vi "Integral timescale and std errors_PN.vi"(0 "uv_bar (m/s)^2":dbl, 1 "Cross-correlation function":dbl[](array[numeric]), 5 "u2v2_bar (m/s)^4":dbl, 7 "T_meas (s)":dbl, 9 "dt (s)":dbl, 11 "integral cut-off":dbl, 12 "integral post-mult":dbl=1.0, 13 "Multiplyer of Timescale to get Independant samples":dbl=2.0) -> (4 "N independent samples":i32, 6 "Integral timescale (s)":dbl, 10 "Std. err in U (m/s)":dbl, 15 "Std. err in uv (m/s^2)":dbl)   [LabVIEW 2016]
uses:
  <vilib>/Analysis/2dsp.llb/Integral Method.ctl
  <vilib>/Analysis/8numeric.llb/1D Numeric Integration.vi
  <vilib>/Analysis/NI_AALPro.lvlib
panel:
  out "Normalised cross-correlation function up to cut-offs":cluster{dbl, "dt (s)":dbl, "Rxy":dbl[]}(graph)
  out "Cross-correlation function (positive signed)":cluster{dbl, "dt (s)":dbl, "Rxy":dbl[]}(graph)
  # "SE_mean is only meaningful in autocorrelation  (i.e. with U = V)"
  # "PN 06/01/2011,\n      01/12/2016"
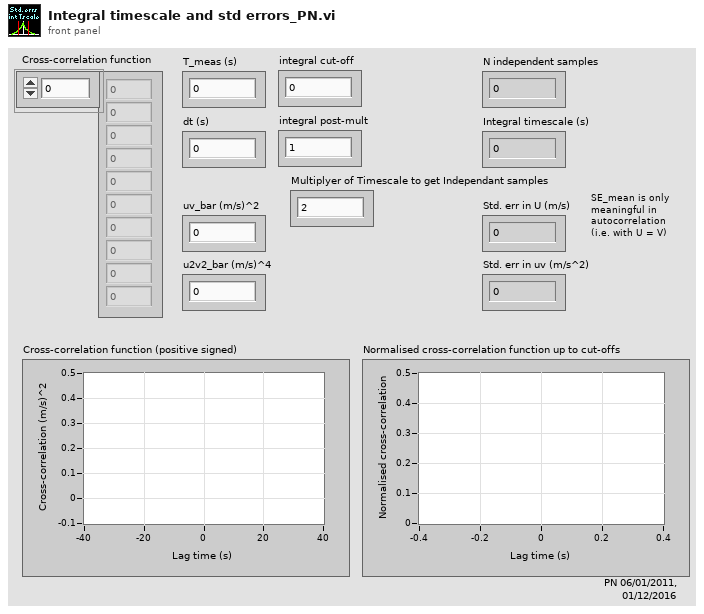
[diagram p1: front panel]
types:
  T1 = typedef "NI_AALPro.lvlib/Integral Method.ctl" = i32
  T2 = cluster{dbl, "dt (s)":dbl, "Cross-correlation function":dbl[]}
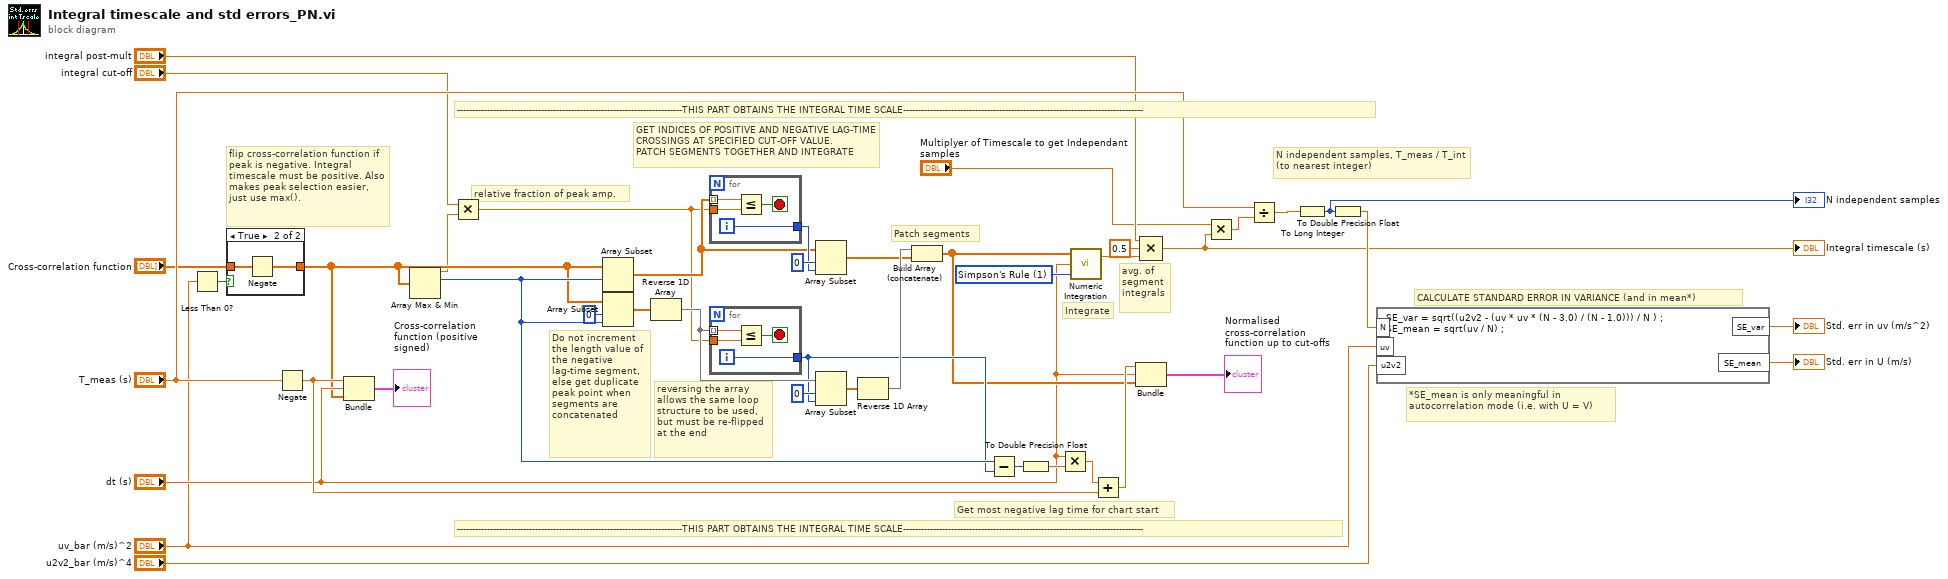
[diagram p0: block diagram]
diagram:
  w42 = T1 1 items=["Trapezoidal Rule", "Simpson's Rule", "Simpson's 3/8 Rule", "Bode Rule"] ("integration method")
  # "flip cross-correlation function if peak is negative. Integral timescale must be positive. Also makes peak selection easier, just use max()."
  # "relative fraction of peak amp."
  # "*SE_mean is only meaningful in autocorrelation mode (i.e. with U = V)"
  # "---------------------------------------------------------------------------THIS PART OBTAINS THE INTEGRAL TIME SCALE--------------------------------------------------------------------------------"
  # "---------------------------------------------------------------------------THIS PART OBTAINS THE INTEGRAL TIME SCALE--------------------------------------------------------------------------------"
  # "Get most negative lag time for chart start"
  # "CALCULATE STANDARD ERROR IN VARIANCE (and in mean*)"
  # "avg. of segment integrals"
  # "Integrate"
  # "Patch segments"
  # "reversing the array allows the same loop structure to be used, but must be re-flipped at the end"
  # "Do not increment the length value of the negative lag-time segment, else get duplicate peak point when segments are concatenated"
  # "N independent samples, T_meas / T_int  (to nearest integer)"
  # "GET INDICES OF POSITIVE AND NEGATIVE LAG-TIME CROSSINGS AT SPECIFIED CUT-OFF VALUE.\nPATCH SEGMENTS TOGETHER AND INTEGRATE"
  n1 = Less Than 0?(x="uv_bar (m/s)^2") -> (x < 0?=w8:bool)
  n2 = case shown="True" w8 {
    tunnel: "Cross-correlation function" -> [w43 w45]
    tunnel: [w43 w44] -> w7
    frame False {
    }
    frame True {
      n3 = Negate(x=w45) -> (-x=w44:dbl[])
    }
  }
  n4 = Negate(x="T_meas (s)") -> (-x=w19:dbl)
  n5 = Bundle(w19, "dt (s)"="dt (s)", "Cross-correlation function"=w7) -> (→"Cross-correlation function (positive signed)":T2)  [unwired: 1 in]
  n6 = Array Max & Min(array=w7) -> (max value=w5:dbl, max index (indices)=w24:i32)  [unwired: 2 out]
  n7 = Multiply(x="integral cut-off", y=w5) -> (x*y=w4:dbl)
  n8 = Array Subset(array=w7, index=w24) -> (w36:dbl[])  [unwired: 1 in]
  n9 = Array Subset(array=w7, index=0, length=w24) -> (w37:dbl[])
  n10 = Reverse 1D Array(array=w37) -> (reversed array=w34:dbl[])
  n11 = for {
    tunnel: w36 -> [w48] mode=indexing
    tunnel: [w49] -> w40
    tunnel: w4 -> [w47]
    i -> [w49]
    stop <- w46 stop-if-true
    n12 = Less Or Equal?(x=w48, y=w47) -> (x <= y?=w46:bool)
  }
  n13 = for {
    tunnel: w34 -> [w52] mode=indexing
    tunnel: [w53] -> w23
    tunnel: w4 -> [w51]
    i -> [w53]
    stop <- w50 stop-if-true
    n14 = Less Or Equal?(x=w52, y=w51) -> (x <= y?=w50:bool)
  }
  n15 = Array Subset(array=w36, index=0, length=w40) -> (w31:dbl[])
  n16 = Array Subset(array=w34, index=0, length=w23) -> (w33:dbl[])
  n17 = Reverse 1D Array(array=w33) -> (reversed array=w32:dbl[])
  n18 = Build Array (concatenate)(w32, w31) -> (w21:dbl[])
  n19 = Subtract(x=w24, y=w23) -> (x-y=w25:i32)
  n20 = To Double Precision Float(number=w25) -> (double precision float=w27:dbl)
  n21 = Multiply(x="dt (s)", y=w27) -> (x*y=w26:dbl)
  n22 = call-poly <vilib>:"Numeric Integration.vi"("integration method"=w42, "dt"="dt (s)", "Input Array"=w21) -> ("result"=w39:dbl)  [unwired: 1 out]
  n23 = Add(x=w26, y=w19) -> (x+y=w22:dbl)
  n24 = Bundle(w22, "dt (s)"="dt (s)", w21) -> (→"Normalised cross-correlation function up to cut-offs":cluster{dbl, "dt (s)":dbl, dbl[]})  [unwired: 1 in]
  n25 = Compound Arithmetic op=MULTIPLY("integral post-mult", 0.5 ("x"), w39) -> (w2:dbl)
  "Integral timescale (s)" <- w2
  n26 = Multiply(x="Multiplyer of Timescale to get Independant samples", y=w2) -> (x*y=w3:dbl)
  n27 = Divide(x="T_meas (s)", y=w3) -> (x/y=w29:dbl)
  n28 = To Long Integer(number=w29) -> (32bit integer=w14:i32)
  "N independent samples" <- w14
  n29 = To Double Precision Float(number=w14) -> (double precision float=w28:dbl)
  n30 = formula code="SE_var = sqrt((u2v2 - (uv * uv * (N - 3.0) / (N - 1.0))) / N ) ;\nSE_mean = sqrt(uv / N) ;"("N"=w28, "u2v2"="u2v2_bar (m/s)^4", "uv"="uv_bar (m/s)^2") -> ("SE_var"=→"Std. err in uv (m/s^2)":dbl, "SE_mean"=→"Std. err in U (m/s)":dbl)
